vi "Test Confluence VIDoc.vi"() -> ()   [LabVIEW 2023]
uses:
  <userlib>/_PetranWay/LabVIEW Confluence API/Source/Confluence/Confluence Connection/Confluence.lvclass
  <userlib>/_PetranWay/LabVIEW Confluence API/Source/Cloud/Confluence Cloud/Confluence Cloud.lvclass
  <vilib>/DMC/VIDoc/Framework/UI Interaction/Progress Bar UI/Progress Bar UI.lvclass
  <userlib>/_PetranWay/LabVIEW Confluence API/Source/Cloud/Confluence Cloud/API/Construct Confluence Cloud From Cache.vi
  <vilib>/DMC/VIDoc/Printers/Confluence/Confluence Printer/VIDoc Printer - Confluence.lvclass
  <vilib>/DMC/VIDoc/Framework/Parsing/Documentation Parser/VIDoc Parser.lvclass
panel:
  in  "Git History?":bool
  in  "Tab Control":enum32{"Use Settings File", "Cloud Connection"}(tab)
  in  "Organization Name":string caption="Organization Name (https://[Organization Name].atlassian.net]"
  in  "Email Address":string
  in  "Top Page ID":string
  in  "Source Root":path
  in  "VIDoc json Settings Path":path
  out "Group":string
  out "Section":string
  out "error out":errorcluster {"code" format="Error %.0f"}
  out "Message":string
  out "Progress Bar":i32(slide) max=28 scale=0.0..7.0
  in  "Abort":bool
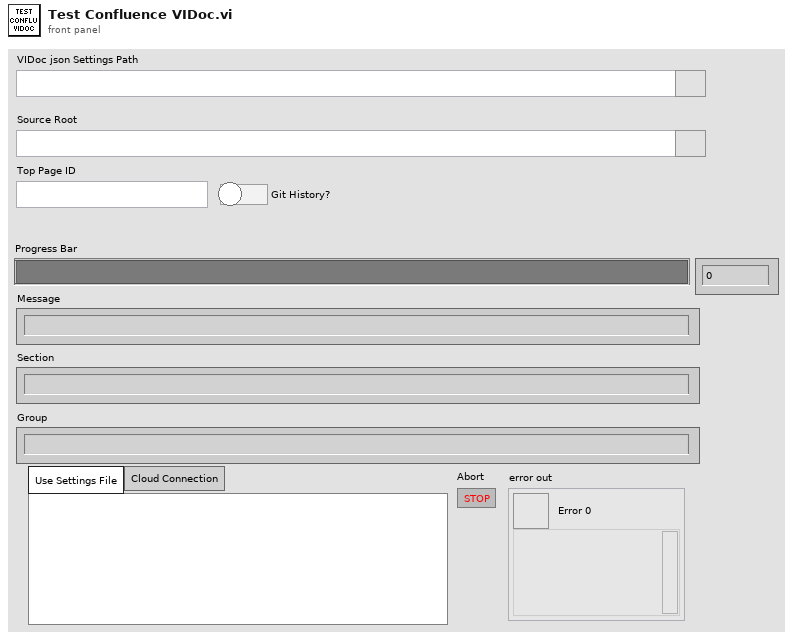
[diagram p1: front panel]
types:
  T1 = cluster{"Progress Max":refnum<user-event>, "Progress Value":refnum<user-event>, "Message":refnum<user-event>, "Stopped":refnum<user-event>, "Section":refnum<user-event>, "Group":refnum<user-event>}
  T2 = typedef "VIDoc Parsing.lvlib/Full Documentation Info.ctl" = cluster{"Projects":refnum<class "Project Documentation.lvclass">[], "Interfaces":refnum<class "Interface Documenation.lvclass">[], "Classes":refnum<class "Class Documentation.lvclass">[], "Libraries":refnum<class "Library Documentation.lvclass">[], "VI Members":refnum<class "GUI Documentation.lvclass">[], "Controls":refnum<class "GUI Documentation.lvclass">[], "LLBs":refnum<class "LLB Documentation.lvclass">[], "Bookmarked Map":map{string, refnum<class "GUI Documentation.lvclass">[]}}
  T3 = typedef "VIDoc Printer - Confluence.lvlib/VIDoc Printer - Confluence.lvclass/File Change Map.ctl" = map{string, cluster{"Timestamp":timestamp, "Commit Hash":string, "Author Name":string, "Branch":string, "Commit Hash URL":string}}
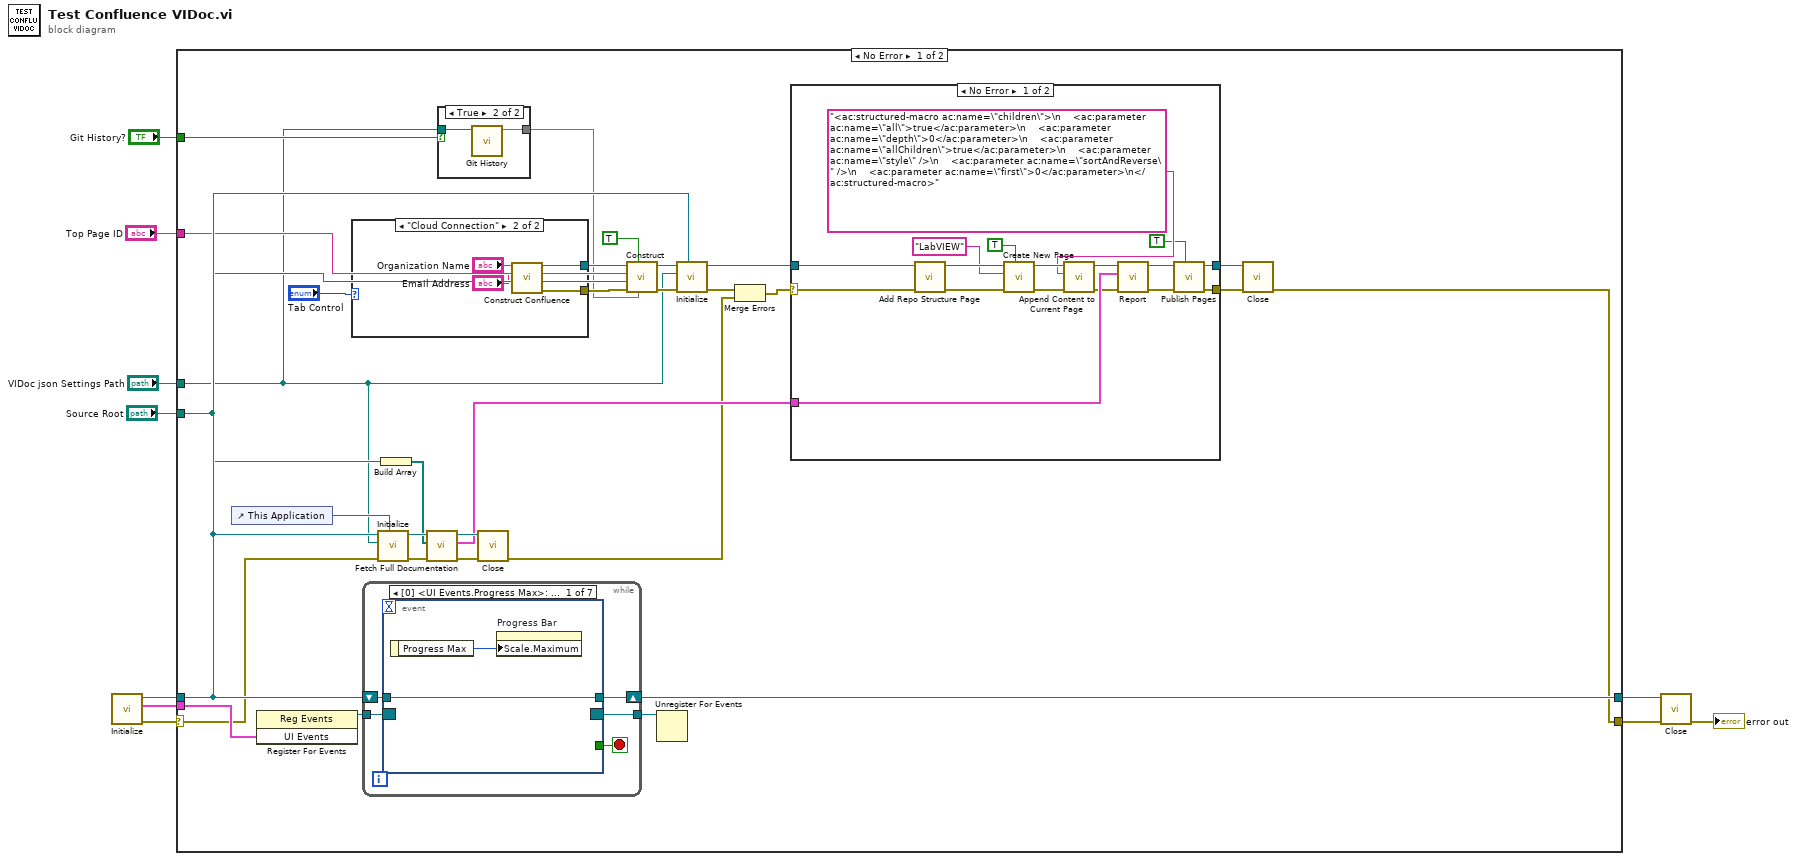
[diagram p0: block diagram]
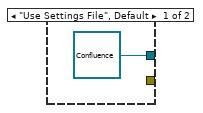
[diagram p3: hidden frame]
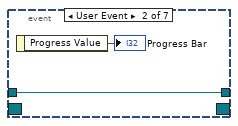
[diagram p5: hidden frame]
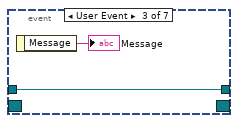
[diagram p6: hidden frame]
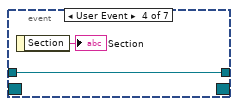
[diagram p7: hidden frame]
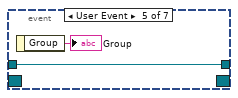
[diagram p8: hidden frame]
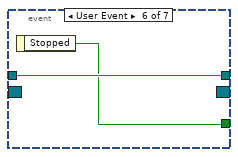
[diagram p9: hidden frame]
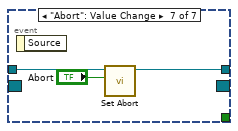
[diagram p10: hidden frame]
diagram:
  n1 = call <vilib>:"Initialize.vi"() -> ("error out"=w7:errorcluster, "UI Events"=w10:T1, "Progress Bar UI Out"=w8:refnum<class "Progress Bar UI.lvclass">)  [unwired: 9 in]
  n2 = case shown="No Error" w7 {
    selector: w7 -> [w29 w89]
    tunnel: w10 -> [w41 _]
    tunnel: [w39 w88] -> w9
    tunnel: w8 -> [w38 w88]
    tunnel: [w33 w89] -> w6
    tunnel: "VIDoc json Settings Path" -> [w12 _]
    tunnel: "Source Root" -> [w28 _]
    tunnel: "Top Page ID" -> [w27 _]
    tunnel: "Git History?" -> [w13 _]
    frame No Error {
      n3 = control-ref of="This Application"() -> (w30:refnum<vi>)
      n4 = register-events(w41) -> (reference out=w40:refnum<event-registration>)  [unwired: 2 in, 1 out]
      n5 = case shown="\"Cloud Connection\"" "Tab Control" {
        tunnel: [refnum<class "Confluence.lvclass"> refnum ("Confluence") w46] -> w16
        tunnel: [_ w45] -> w15
        frame "Use Settings File", Default {
        }
        frame "Cloud Connection" {
          n6 = call-poly <userlib>:"Construct Confluence.vi"("Organization Name (https://[Organization Name].atlassian.net]"="Organization Name", "Email Address"="Email Address") -> ("Confluence Cloud out"=w46:refnum<class "Confluence Cloud.lvclass">, "error out"=w45:errorcluster)  [unwired: 10 in, 2 out]
        }
      }
      n7 = while {
        tunnel: w40 -> [w72]
        shift-right: [w70] -> w39
        shift-left: w38 -> [w71]
        tunnel: [w68] -> w26
        stop <- w69 stop-if-true
        n8 = event shown="[0] <UI Events.Progress Max>: User Event" {
          selector: w72 -> [_ _ _ _ _ _ _]
          dyn-events: [_ _ _ _ _ _ _] -> w68
          timeout: _ -> [_ _ _ _ _ _ _]
          tunnel: w71 -> [w74 w76 w78 w80 w82 w84 w86]
          tunnel: [w74 w76 w78 w80 w82 w84 w87] -> w70
          tunnel: [_ _ _ _ _ w83 _] -> w69
          event User Event {
            n9 = event-data() -> ("Progress Max"=w73:i32)  [unwired: 1 in]
            n10 = property on="Progress Bar" class="Slide (strict)"("Scale.Maximum"=w73) -> ()  [unwired: 2 in, 2 out]
          }
          event User Event {
            n11 = event-data() -> ("Progress Value"=→"Progress Bar":i32)  [unwired: 1 in]
          }
          event User Event {
            n12 = event-data() -> ("Message"=→"Message":string)  [unwired: 1 in]
          }
          event User Event {
            n13 = event-data() -> ("Section"=→"Section":string)  [unwired: 1 in]
          }
          event User Event {
            n14 = event-data() -> ("Group"=→"Group":string)  [unwired: 1 in]
          }
          event User Event {
            n15 = event-data() -> ("Stopped"=w83:bool)  [unwired: 1 in]
          }
          event "Abort": Value Change {
            n16 = event-data() -> ()  [unwired: 1 in, 1 out]
            n17 = call <vilib>:"Set Abort.vi"("Abort?"="Abort", "Progress Bar UI In"=w86) -> ("Progress Bar UI Out"=w87:refnum<class "Progress Bar UI.lvclass">)  [unwired: 8 in, 1 out]
          }
        }
      }
      n18 = call <vilib>:"Initialize.vi"("App Reference (This Application)"=w30, "error in (no error)"=w29, "Settings Path"=w12, "UI Interaction"=w38) -> ("error out"=w37:errorcluster, "VIDoc Parser Out"=w36:refnum<class "VIDoc Parser.lvclass">)  [unwired: 6 in]
      n19 = Build Array(w28) -> (w31:path[])
      n20 = call <vilib>:"Fetch Full Documentation.vi"("error in (no error)"=w37, "File Paths"=w31, "VIDoc Parser In"=w36) -> ("error out"=w34:errorcluster, "Full Documentation"=w32:T2, "VIDoc Parser Out"=w35:refnum<class "VIDoc Parser.lvclass">)  [unwired: 6 in]
      n21 = case shown="True" w13 {
        tunnel: [_ w43] -> w11
        tunnel: w12 -> [_ w42]
        frame False {
        }
        frame True {
          n22 = call "Git History.vi"("Working Directory"=w42) -> ("File Change Map"=w43:T3)  [unwired: 9 in, 1 out]
        }
      }
      n23 = call <vilib>:"Close.vi"("error in (no error)"=w34, "VIDoc Parser In"=w35) -> ("error out"=w17:errorcluster)  [unwired: 9 in]
      n24 = call <vilib>:"Construct.vi"("File Change Map"=w11, "Bulk Attachments? (T)"=TRUE, "error in (no error)"=w15, "Working Directory"=w28, "Top Page ID"=w27, "Confluence"=w16) -> ("error out"=w25:errorcluster, "VIDoc Printer - Confluence Out"=w24:refnum<class "VIDoc Printer - Confluence.lvclass">)  [unwired: 4 in]
      n25 = Unregister For Events(event registration refnum=w26) -> ()  [unwired: 1 in, 1 out]
      n26 = call-dynamic <vilib>:"Initialize.vi"("UI Interaction"=w38, "error in (no error)"=w25, "Settings Path"=w12, "VIDoc Printer - Confluence In"=w24) -> ("error out"=w23:errorcluster, "VIDoc Printer - Confluence Out"=w22:refnum<class "VIDoc Printer - Confluence.lvclass">)  [unwired: 6 in]
      n27 = Merge Errors(w23, w17) -> (w18:errorcluster)
      n28 = case shown="No Error" w18 {
        selector: w18 -> [w64 w66]
        tunnel: w32 -> [w65 _]
        tunnel: w22 -> [w63 w67]
        tunnel: [w62 w66] -> w20
        tunnel: [w61 w67] -> w19
        frame No Error {
          n29 = call <vilib>:"Add Repo Structure Page.vi"("error in (no error)"=w64, "VIDoc Printer - Confluence In"=w63) -> ("error out"=w58:errorcluster, "VIDoc Printer - Confluence Out"=w57:refnum<class "VIDoc Printer - Confluence.lvclass">)  [unwired: 8 in]
          n30 = call <vilib>:"Create New Page.vi"("Update Current Page (F)"=TRUE, "error in (no error)"=w58, "Name"="LabVIEW", "VIDoc Printer - Confluence In"=w57) -> ("error out"=w52:errorcluster, "VIDoc Printer - Confluence Out"=w54:refnum<class "VIDoc Printer - Confluence.lvclass">)  [unwired: 4 in, 2 out]
          n31 = call <vilib>:"Append Content to Current Page.vi"("error in (no error)"=w52, "Content"="<ac:structured-macro ac:name=\"children\">\n    <ac:parameter ac:name=\"all\">true</ac:parameter>\n    <ac:parameter ac:name=\"depth\">0</ac:parameter>\n    <ac:parameter ac:name=\"allChildren\">true</ac:parameter>\n    <ac:parameter ac:name=\"style\" />\n    <ac:parameter ac:name=\"sortAndReverse\" />\n    <ac:parameter ac:name=\"first\">0</ac:parameter>\n</ac:structured-macro>", "VIDoc Printer - Confluence In"=w54) -> ("error out"=w51:errorcluster, "VIDoc Printer - Confluence Out"=w53:refnum<class "VIDoc Printer - Confluence.lvclass">)  [unwired: 7 in]
          n32 = call-dynamic "Report.vi"("error in (no error)"=w51, "Full Documentation"=w65, "VIDoc Printer In"=w53) -> ("error out"=w60:errorcluster, "VIDoc Printer Out"=w59:refnum<class "VIDoc Printer - Confluence.lvclass">)  [unwired: 7 in]
          n33 = call <vilib>:"Publish Pages.vi"("Parallel?"=TRUE, "error in (no error)"=w60, "VIDoc Printer - Confluence In"=w59) -> ("error out"=w62:errorcluster, "VIDoc Printer - Confluence Out"=w61:refnum<class "VIDoc Printer - Confluence.lvclass">)  [unwired: 7 in]
        }
        frame Error {
        }
      }
      n34 = call-dynamic <vilib>:"Close.vi"("error in (no error)"=w20, "VIDoc Printer - Confluence In"=w19) -> ("error out"=w33:errorcluster)  [unwired: 9 in]
    }
    frame Error {
    }
  }
  n35 = call <vilib>:"Close.vi"("error in (no error)"=w6, "Progress Bar UI In"=w9) -> ("error out"=→"error out":errorcluster)  [unwired: 9 in]
